vi "Class Name.vi"(8 "error in (no error)":errorcluster, 11 "Scale in":refnum<class "Scale.lvclass">) -> (0 "error out":errorcluster, 2 "Class Name":string, 3 "Scale out":refnum<class "Scale.lvclass">)   [LabVIEW 2021, in "Scale.lvclass"]
uses:
  Scale.lvclass
  Scale.lvclass/Scale.ctl
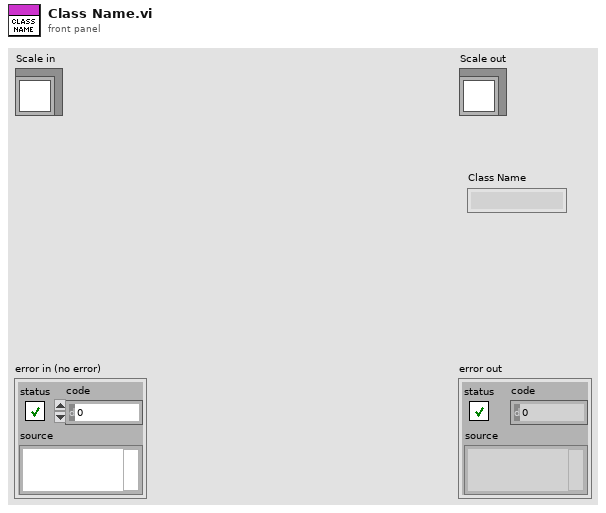
[diagram p1: front panel]
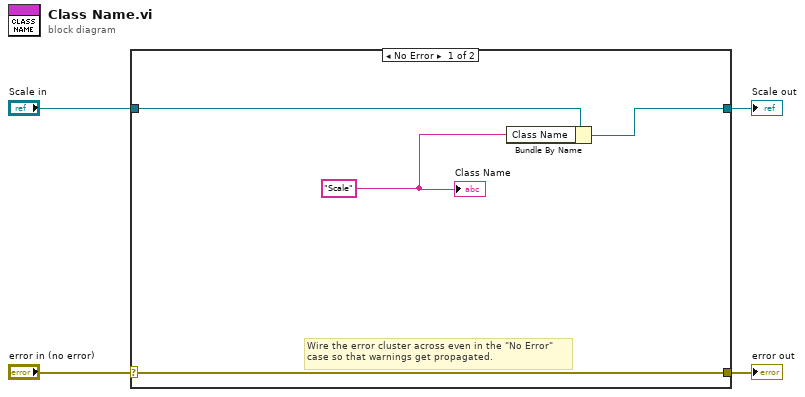
[diagram p0: block diagram]
diagram:
  n1 = case shown="No Error" "error in (no error)" {
    selector: "error in (no error)" -> [w8 w10]
    tunnel: [w8 w10] -> w3
    tunnel: [w7 w9] -> w1
    tunnel: "Scale in" -> [w6 w9]
    frame No Error {
      w5 = "Scale"
      # "Wire the error cluster across even in the \"No Error\"\ncase so that warnings get propagated."
      n2 = Bundle By Name(cluster=w6, "Class Name"=w5) -> (w7:refnum<class "Scale.lvclass">)
      "Class Name" <- w5
    }
    frame Error {
    }
  }
  "error out" <- w3
  "Scale out" <- w1
